vi "FPGA Phasor Measurement for P Class (50 Hz).vi"(0 "signal in":fxp<+/-,24,1>, 1 "number of channels":T2=1 items=["1"=1, "2"=2, "3"=3, "4"=4, "5"=5, "6"=6, "7"=7, "8"=8, "9"=9, "10"=10, "11"=11, "12"=12, "13"=13, "14"=14, "15"=15, "16"=16], 5 "timestamp [s]":fxp<+,64,32>, 7 "reference channel index (0)":u8, 9 "input valid? (T)":bool=TRUE, 12 "ready for output? (T)":bool=TRUE) -> (4 "output data":T1 {"timestamp [s]" format="%#.6g"; "phase [pi]" format="%#.6g"}, 10 "output valid?":bool, 14 "ready for input?":bool, 15 "error":i32)   [LabVIEW 2014, in "NI_EP_PMU_FPGA.lvlib"]
doc: "Calculates the instantaneous magnitude, phase, and frequency values of the fundamental frequency component as defined in the P class of performance in IEEE Std C37.118.1-2011. This VI resamples even-time-spaced voltage and current signals into even-angle-spaced signals. The input signals must have a sample rate of 50 kHz. The output rate is 25 samples per cycle. You must manually select the polymorphic instance to use."
uses:
  <vilib>/addons/Electrical Power/PMU/NI_EP_PMU_FPGA.lvlib
  <vilib>/addons/Electrical Power/PQ/Resampling/FPGA/subVIs/fpga_NofCH.ctl
  <vilib>/addons/Electrical Power/PQ/Resampling/NI_EP_Resample_FPGA.lvlib
  <vilib>/addons/Electrical Power/PMU/FPGA/subVIs/fpga_OutputDataType.ctl
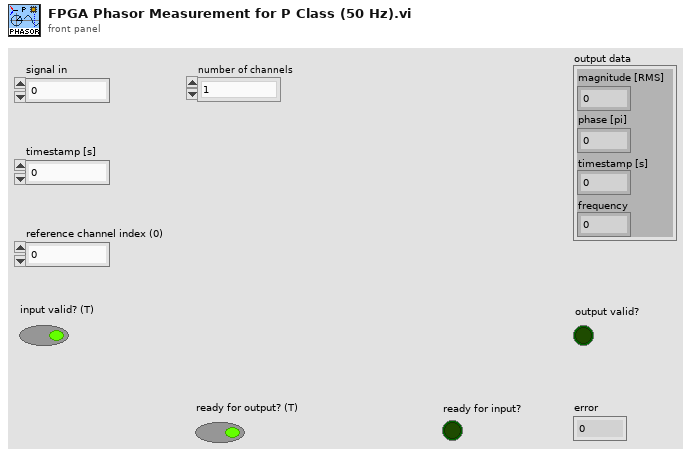
[diagram p1: front panel]
types:
  T1 = typedef "NI_EP_PMU_FPGA.lvlib/fpga_OutputDataType.ctl" = cluster{"magnitude [RMS]":fxp<+,32,6>, "phase [pi]":fxp<+/-,32,2>, "timestamp [s]":fxp<+,64,32>, "frequency":fxp<+,32,8>}
  T2 = typedef "NI_EP_Resample_FPGA.lvlib/fpga_NofCH.ctl" = u8
  T3 = typedef "NI_EP_Resample_FPGA.lvlib/fpga_Resampled.ctl" = cluster{"signal":fxp<+/-,32,3>, "timestamp [s]":fxp<+,64,32>, "frequency":fxp<+,32,8>}
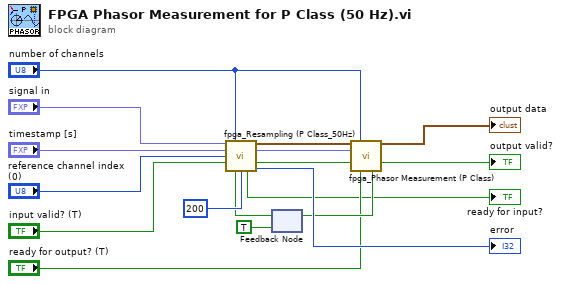
[diagram p0: block diagram]
diagram:
  n1 = feedback #1(TRUE ("ready for input")) -> (w10:bool)
  n2 = call <vilib>:"fpga_Resampling (P Class_50Hz).vi"("signal in"="signal in", "number of channels"="number of channels", "timestamp [s]"="timestamp [s]", "reference channel index"="reference channel index (0)", "input valid? (T)"="input valid? (T)", "ready for output? (T)"=w10, "samples per cycle"=u16 200) -> ("resampled data"=w8:T3, "freq time difference [s]"=w3:fxp<+,18,-4>, "output valid?"=w2:bool, "ready for input"=→"ready for input?":bool, "error"=→"error":i32)  [unwired: 4 in]
  n3 = call <vilib>:"fpga_Phasor Measurement (P Class).vi"("resampled data"=w8, "number of channels"="number of channels", "freq time difference [s]"=w3, "input valid? (T)"=w2, "ready for output? (T)"="ready for output? (T)") -> ("output data"=→"output data":T1, "output valid?"=→"output valid?":bool, "ready for input?"=w9:bool)  [unwired: 8 in]
  n4 = feedback-in #1(w9) -> ()
